vi "Word transmission.vi"() -> ()   [LabVIEW 2020]
panel:
  out "Batch Length":i32
  out "Actual Bitrate kHz 2":i32=1000
  in  "SDI":u64[](array[numeric]) format="%.0x"
  out "dup Cheetah Handle":i32
  out "Total Shifted Out":i32
  out "Actual Bitrate kHz":i32=1000
  out "error out":errorcluster
  in  "Rds per Sec":dbl=2000.0 max=2000000000.0
  out "SDO":u64[](array[numeric]) format="%x"
  in  "SCLK (kHz)":i32=2000 min=0
  out "Cheetah Handle":i32
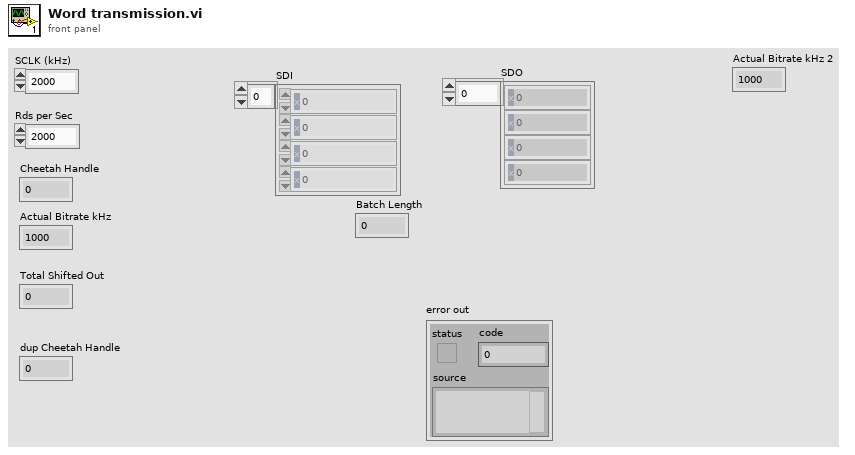
[diagram p1: front panel]
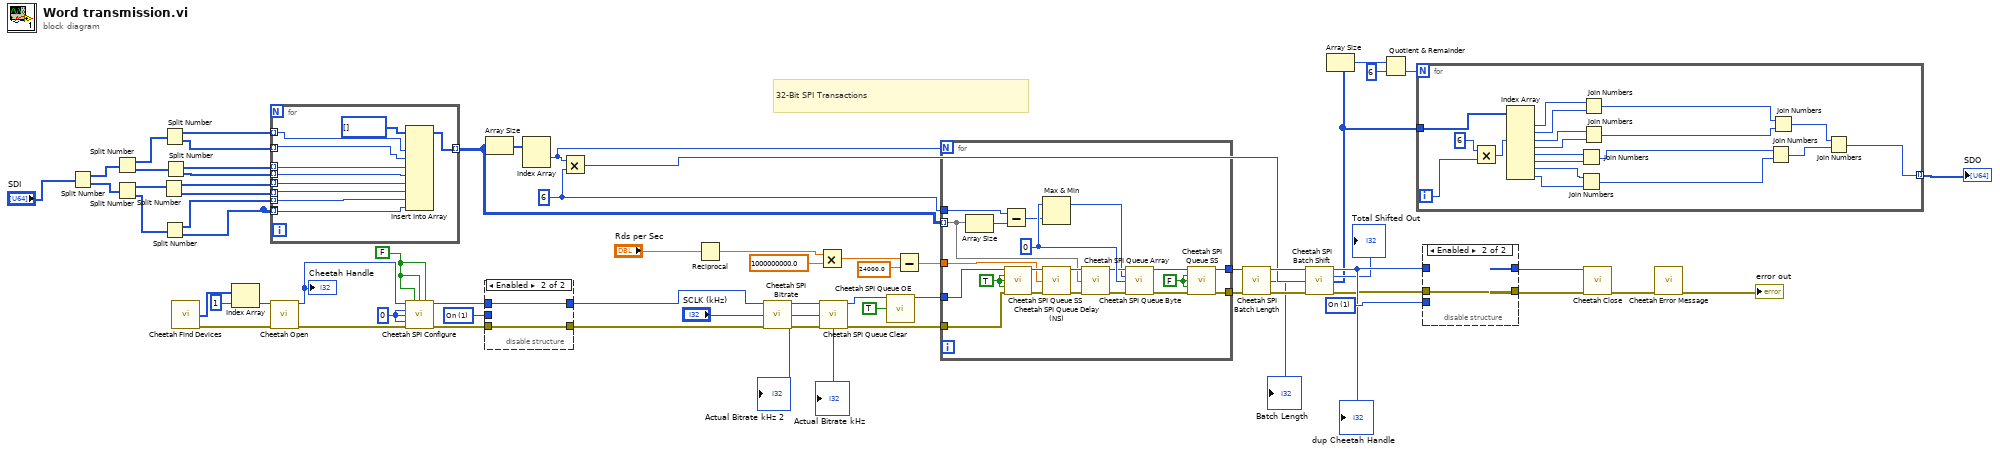
[diagram p0: block diagram]
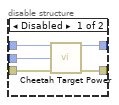
[diagram p2: hidden frame]
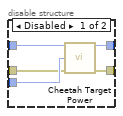
[diagram p3: hidden frame]
diagram:
  w20 = 6 ("y")
  w45 = u16 1 items=["Off", "On", "Query"] ("Requested Configuration (2: Query)")
  w46 = u16 1 items=["Off", "On", "Query"] ("Requested Configuration (2: Query)")
  w61 = FALSE
  w63 = 0
  # "32-Bit SPI Transactions"
  n1 = Split Number(x="SDI") -> (hi(x)=w31:u32[], lo(x)=w30:u32[])
  n2 = Split Number(x=w31) -> (hi(x)=w7:u16[], lo(x)=w6:u16[])
  n3 = Split Number(x=w30) -> (hi(x)=w10:u16[], lo(x)=w9:u16[])
  n4 = Split Number(x=w10) -> (hi(x)=w14:u8[], lo(x)=w13:u8[])
  n5 = Split Number(x=w7) -> (hi(x)=w5:u8[], lo(x)=w4:u8[])
  n6 = Split Number(x=w9) -> (hi(x)=w12:u8[], lo(x)=w11:u8[])
  n7 = Split Number(x=w6) -> (hi(x)=w3:u8[], lo(x)=w2:u8[])
  n8 = call <instrlib>:"Cheetah Find Devices.vi"() -> ("Ports"=w64:u16[], "error out"=w60:errorcluster)  [unwired: 13 in, 1 out]
  n9 = Index Array(array=w64, index=1) -> (element=w52:u16)
  n10 = for {
    tunnel: w14 -> [w75] mode=indexing
    tunnel: [w74] -> w29 mode=indexing
    tunnel: w12 -> [w72] mode=indexing
    tunnel: w11 -> [_] mode=indexing
    tunnel: w11 -> [w71] mode=indexing
    tunnel: w13 -> [w70] mode=indexing
    tunnel: w5 -> [w69] mode=indexing
    tunnel: w4 -> [w68] mode=indexing
    tunnel: w3 -> [w67] mode=indexing
    tunnel: w2 -> [w66] mode=indexing
    n11 = Insert Into Array(array=u8[] [], new element #1=w69, new element #2=w68, new element #3=w67, new element #4=w66, new element #5=w75, new element #6=w70, new element #7=w72, new element #8=w71) -> (w74:u8[])  [unwired: 1 in]
  }
  n12 = call <instrlib>:"Cheetah Open.vi"("Port Number (0)"=w52, "error in (no error)"=w60) -> ("Cheetah Handle"=w57:i32, "error out"=w59:errorcluster)  [unwired: 12 in]
  "Cheetah Handle" <- w57
  n13 = call <instrlib>:"Cheetah SPI Configure.vi"("Cheetah Handle"=w57, "SS0 Active High? (False)"=w61, "SS1 Active High? (False)"=w61, "SS2 Active High? (False)"=w61, "Polarity (0: Rising/Falling)"=w63, "Phase (0: Sample/Setup)"=w63, "Bitorder (0: MSB)"=w63, "error in (no error)"=w59) -> ("dup Cheetah Handle"=w56:i32, "error out"=w58:errorcluster)  [unwired: 6 in]
  n14 = disable-structure shown="Enabled" {
    disable-tunnel: w58 -> [w80 w81]
    disable-tunnel: w56 -> [w79 w82]
    disable-tunnel: [w78 w81] -> w55
    disable-tunnel: [w77 w82] -> w53
    disable-tunnel: w45 -> [w76 _]
    frame Disabled {
      n15 = call <instrlib>:"Cheetah Target Power.vi"("Cheetah Handle"=w79, "Requested Configuration (2: Query)"=w76, "error in (no error)"=w80) -> ("dup Cheetah Handle"=w77:i32, "error out"=w78:errorcluster)  [unwired: 10 in, 1 out]
    }
    frame Enabled {
    }
  }
  n16 = Array Size(array=w29) -> (size(s)=w44:i32[])
  n17 = Index Array(array=w44) -> (element #1=w16:i32)  [unwired: 2 in, 1 out]
  n18 = Multiply(x=w16, y=w20) -> (x*y=w15:i32)
  n19 = Reciprocal(x="Rds per Sec") -> (1/x=w22:dbl)
  n20 = call <instrlib>:"Cheetah SPI Bitrate.vi"("Cheetah Handle"=w53, "Requested Bitrate kHz (1000)"="SCLK (kHz)", "error in (no error)"=w55) -> ("dup Cheetah Handle"=w51:i32, "Actual Bitrate kHz"=→"Actual Bitrate kHz" →"Actual Bitrate kHz 2":i32, "error out"=w50:errorcluster)  [unwired: 10 in]
  n21 = Multiply(x=w22, y=1000000000.0) -> (x*y=w25:dbl)
  n22 = call <instrlib>:"Cheetah SPI Queue Clear.vi"("Cheetah Handle"=w51, "error in (no error)"=w50) -> ("dup Cheetah Handle"=w43:i32, "error out"=w62:errorcluster)  [unwired: 12 in]
  n23 = call <instrlib>:"Cheetah SPI Queue OE.vi"("Cheetah Handle"=w43, "Output Enable (on)"=TRUE) -> ("dup Cheetah Handle"=w42:i32)  [unwired: 12 in, 1 out]
  n24 = Subtract(x=w25, y=24000.0) -> (x-y=w23:dbl)
  n25 = for {
    N: w16 -> [_]
    tunnel: w62 -> [w89]
    tunnel: w42 -> [w90]
    tunnel: w29 -> [w91] mode=indexing
    tunnel: [w88] -> w40
    tunnel: [w87] -> w39
    tunnel: w23 -> [w84]
    tunnel: w20 -> [w85]
    w95 = FALSE
    w98 = 0
    w86 = TRUE
    n26 = Array Size(array=w91) -> (size(s)=w92:i32)
    n27 = Subtract(x=w85, y=w92) -> (x-y=w96:i32)
    n28 = call <instrlib>:"Cheetah SPI Queue SS.vi"("Cheetah Handle"=w90, "SS0 Assert? (True)"=w86, "SS1 Assert? (True)"=w86, "SS2 Assert? (True)"=w86, "error in (no error)"=w89) -> ("dup Cheetah Handle"=w103:i32, "error out"=w102:errorcluster)  [unwired: 9 in]
    n29 = Max & Min(x=w98, y=w96) -> (max(x,y)=w83:i32)  [unwired: 1 out]
    n30 = call <instrlib>:"Cheetah SPI Queue Delay (NS).vi"("Cheetah Handle"=w103, "Delay NS (1000)"=w84, "error in (no error)"=w102) -> ("dup Cheetah Handle"=w101:i32, "error out"=w100:errorcluster)  [unwired: 10 in, 1 out]
    n31 = call <instrlib>:"Cheetah SPI Queue Array.vi"("Cheetah Handle"=w101, "Data Out (none)"=w91, "error in (no error)"=w100) -> ("dup Cheetah Handle"=w97:i32, "error out"=w99:errorcluster)  [unwired: 11 in]
    n32 = call <instrlib>:"Cheetah SPI Queue Byte.vi"("Cheetah Handle"=w97, "Byte Count (1)"=w83, "Byte Value (0x00)"=w98, "error in (no error)"=w99) -> ("dup Cheetah Handle"=w94:i32, "error out"=w93:errorcluster)  [unwired: 10 in]
    n33 = call <instrlib>:"Cheetah SPI Queue SS.vi"("Cheetah Handle"=w94, "SS0 Assert? (True)"=w95, "SS1 Assert? (True)"=w95, "SS2 Assert? (True)"=w95, "error in (no error)"=w93) -> ("dup Cheetah Handle"=w87:i32, "error out"=w88:errorcluster)  [unwired: 9 in]
  }
  n34 = call <instrlib>:"Cheetah SPI Batch Length.vi"("Cheetah Handle"=w39, "error in (no error)"=w40) -> ("dup Cheetah Handle"=w38:i32, "Batch Length"=→"Batch Length":i32, "error out"=w37:errorcluster)  [unwired: 11 in]
  n35 = call <instrlib>:"Cheetah SPI Batch Shift.vi"("Cheetah Handle"=w38, "Max Bytes to Retrieve (256)"=w15, "error in (no error)"=w37) -> ("dup Cheetah Handle"=w36:i32, "Total Shifted Out"=→"Total Shifted Out":i32, "Data In"=w17:u8[], "error out"=w28:errorcluster)  [unwired: 9 in]
  "dup Cheetah Handle" <- w36
  n36 = Array Size(array=w17) -> (size(s)=w35:i32)
  n37 = Quotient & Remainder(x=w35, y=6) -> (floor(x/y)=w33:i32)  [unwired: 1 out]
  n38 = for {
    N: w33 -> [_]
    tunnel: w17 -> [w121]
    tunnel: [w118] -> w32 mode=indexing
    i -> [w117]
    n39 = Multiply(x=6, y=w117) -> (x*y=w119:i32)
    n40 = Index Array(array=w121, index #3=w119) -> (element #1=w107:u8, element #2=w106:u8, element #3=w105:u8, element #4=w104:u8, element #5=w116:u8, element #6=w115:u8, element #7=w114:u8, element #8=w113:u8)  [unwired: 7 in]
    n41 = Join Numbers(hi=w116, lo=w115) -> ((hi.lo)=w112:u16)
    n42 = Join Numbers(hi=w114, lo=w113) -> ((hi.lo)=w111:u16)
    n43 = Join Numbers(hi=w107, lo=w106) -> ((hi.lo)=w110:u16)
    n44 = Join Numbers(hi=w105, lo=w104) -> ((hi.lo)=w109:u16)
    n45 = Join Numbers(hi=w112, lo=w111) -> ((hi.lo)=w122:u32)
    n46 = Join Numbers(hi=w110, lo=w109) -> ((hi.lo)=w108:u32)
    n47 = Join Numbers(hi=w108, lo=w122) -> ((hi.lo)=w118:u64)
  }
  "SDO" <- w32
  n48 = disable-structure shown="Enabled" {
    disable-tunnel: [w127 _] -> w49
    disable-tunnel: [w126 w128] -> w48
    disable-tunnel: w46 -> [w125 _]
    disable-tunnel: w36 -> [w124 _]
    disable-tunnel: w28 -> [w123 w128]
    frame Disabled {
      n49 = call <instrlib>:"Cheetah Target Power.vi"("Cheetah Handle"=w124, "Requested Configuration (2: Query)"=w125, "error in (no error)"=w123) -> ("dup Cheetah Handle"=w127:i32, "error out"=w126:errorcluster)  [unwired: 10 in, 1 out]
    }
    frame Enabled {
    }
  }
  n50 = call <instrlib>:"Cheetah Close.vi"("Cheetah Handle"=w49, "error in (no error)"=w48) -> ("error out"=w47:errorcluster)  [unwired: 12 in, 1 out]
  n51 = call <instrlib>:"Cheetah Error Message.vi"("error in (no error)"=w47) -> ("error out"=→"error out":errorcluster)  [unwired: 10 in, 4 out]
